vi "Object by Type Key.vi"(11 "Object In":refnum<class>) -> (2 "Object Type Key":string, 3 "Object":refnum<class>)   [LabVIEW 2020, in "HTTP Server.lvlib" / "Values.lvclass"]
uses:
  Values.lvclass
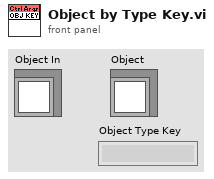
[diagram p1: front panel]
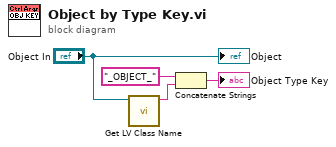
[diagram p0: block diagram]
diagram:
  n1 = call <vilib>:"Get LV Class Name.vi"("object"="Object In") -> ("class name"=w4:string)  [unwired: 9 in, 1 out]
  n2 = Concatenate Strings("_OBJECT_" ("string"), w4) -> (→"Object Type Key":string)
  "Object" <- "Object In"
